vi "主板电池信息配置.vi"(2 "电池信息查看":string[][](table)) -> (0 "输出数组":string[][](array[string]), 1 "布尔":bool=TRUE)   [LabVIEW 2013]
panel:
  in  "整车CAN测试":bool
  in  "电池信息":T1
  in  "停止":bool
  in  "确定":bool
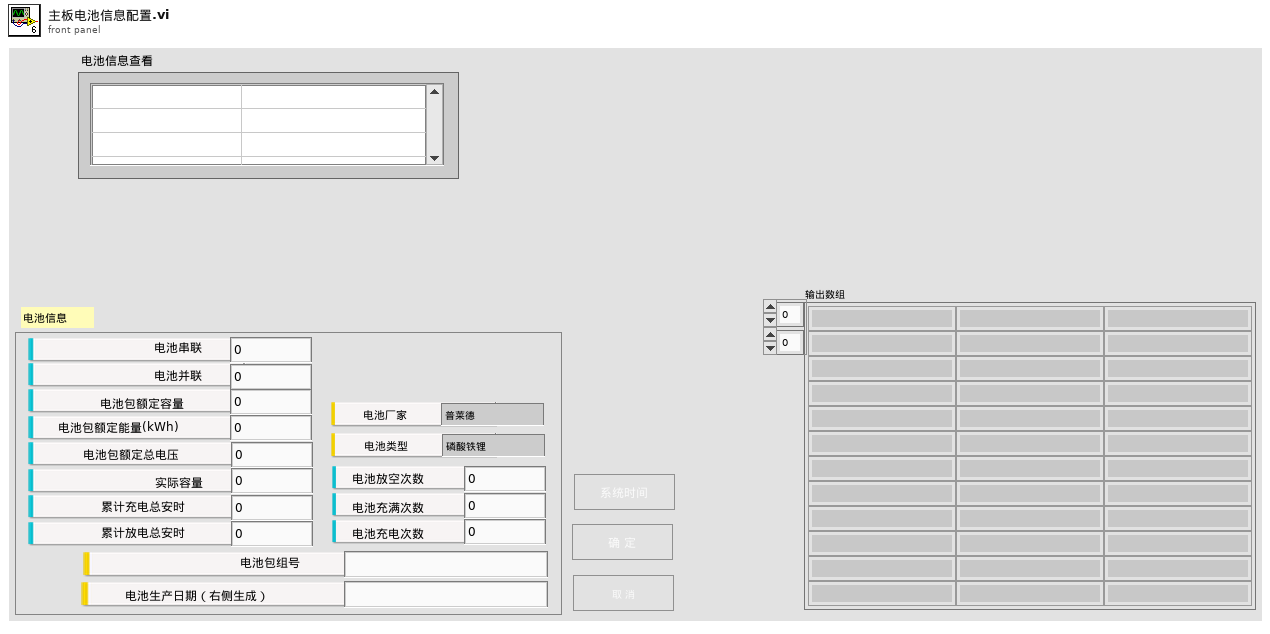
[diagram p1: front panel]
types:
  T1 = cluster{"电池串联":dbl, "电池并联":dbl, "电池包额定容量":dbl, "电池包额定能量(kWh)":dbl, "电池包额定总电压":dbl, "实际容量":dbl, "电池厂家":enum16{"普莱德", "盟固利", "CALB", "力神", "波士顿", "BAK"}, "电池类型":enum16{"磷酸铁锂", "锰酸锂", "三元材料", "铅酸", "镍氢", "钴酸锂", "聚合物锂离子", "钛酸锂", "其他电池"}, "累计充电总安时":dbl, "累计放电总安时":dbl, "电池放空次数":dbl, "电池充满次数":dbl, "电池充电次数":dbl, "电池生产日期（右侧生成）":string, "电池包组号":string}
  T2 = enum16{"磷酸铁锂", "锰酸锂", "三元材料", "铅酸", "镍氢", "钴酸锂", "聚合物锂离子", "钛酸锂", "其他电池"}
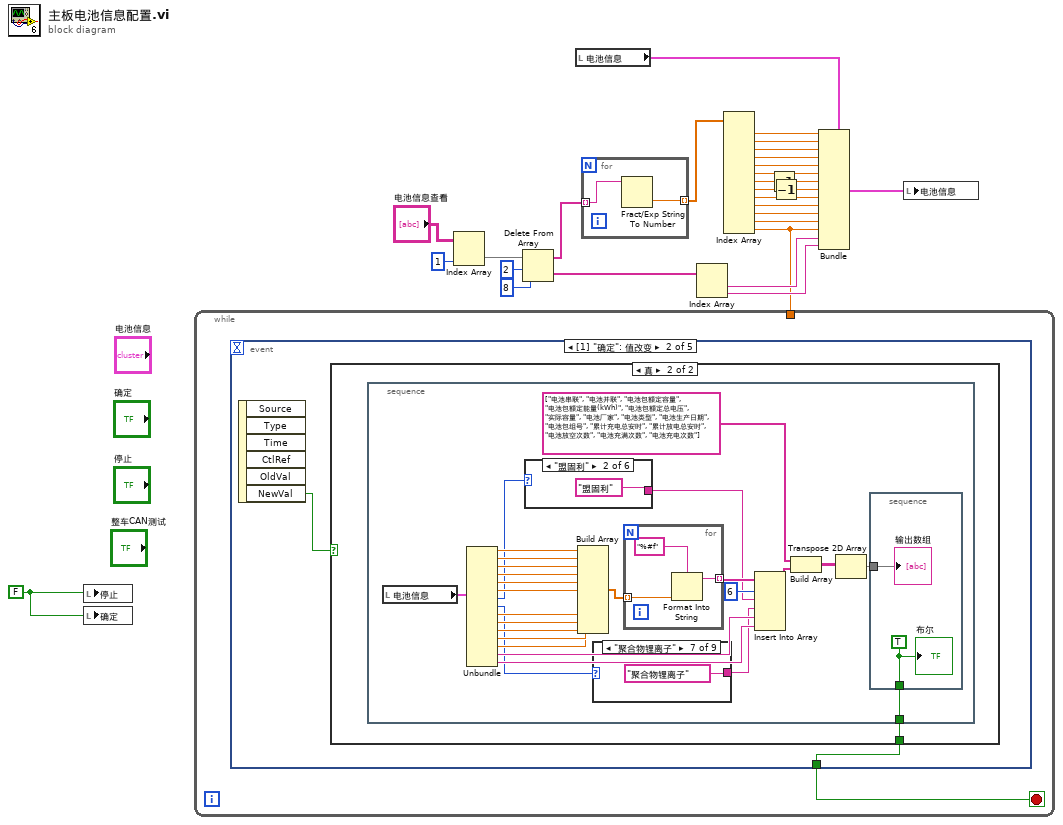
[diagram p0: block diagram]
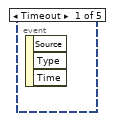
[diagram p2: hidden frame]
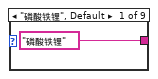
[diagram p4: hidden frame]
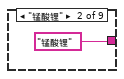
[diagram p5: hidden frame]
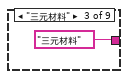
[diagram p6: hidden frame]
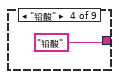
[diagram p7: hidden frame]
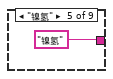
[diagram p8: hidden frame]
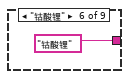
[diagram p9: hidden frame]
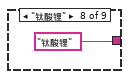
[diagram p10: hidden frame]
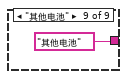
[diagram p11: hidden frame]
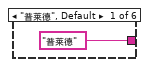
[diagram p12: hidden frame]
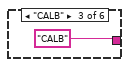
[diagram p13: hidden frame]
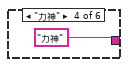
[diagram p14: hidden frame]
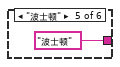
[diagram p15: hidden frame]
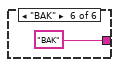
[diagram p16: hidden frame]
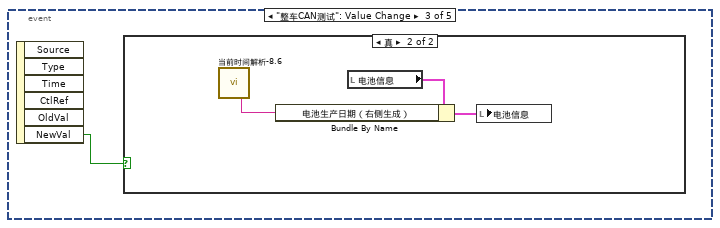
[diagram p17: hidden frame]
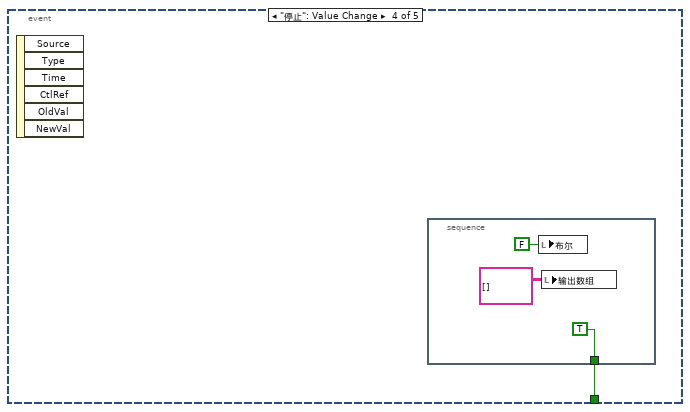
[diagram p19: hidden frame]
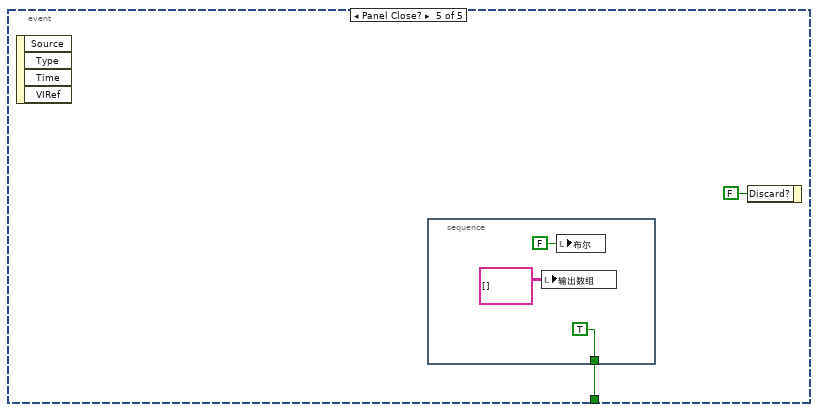
[diagram p20: hidden frame]
diagram:
  w28 = FALSE ("取消按钮")
  n1 = local write "停止"(w28) -> ()
  n2 = local write "确定"(w28) -> ()
  n3 = Index Array(array="电池信息查看", index (col)=1 ("禁用的索引 (列)")) -> (element=w25:string[])  [unwired: 1 in]
  n4 = Delete From Array(array=w25, length=2 ("长度"), index=8 ("索引")) -> (deleted portion=w19:string[], array with subset deleted=w22:string[])
  n5 = local read "电池信息"() -> (w21:T1)
  n6 = for {
    tunnel: w22 -> [w30] mode=indexing
    tunnel: [w29] -> w16 mode=indexing
    n7 = Fract/Exp String To Number(string=w30) -> (number=w29:dbl)  [unwired: 3 in, 1 out]
  }
  n8 = Index Array(array=w19) -> (element #1=w18:string, element #2=w17:string)  [unwired: 2 in]
  n9 = Index Array(array=w16) -> (element #1=w15:dbl, element #2=w14:dbl, element #3=w13:dbl, element #4=w12:dbl, element #5=w11:dbl, element #6=w10:dbl, element #7=w9:dbl, element #8=w8:dbl, element #9=w7:dbl, element #10=w6:dbl, element #11=w5:dbl, element #12=w4:dbl, element #13=w3:dbl)  [unwired: 13 in]
  n10 = while {
    tunnel: w3 -> [_]
    stop <- w31 stop-if-true
    n11 = event shown="[1] \"确定\": 值改变" {
      selector: _ -> [_ _ _ _ _]
      dyn-events: _ -> [_ _ _ _ _]
      timeout: _ -> [_ _ _ _ _]
      tunnel: [_ w32 _ w85 w90] -> w31
      event Timeout {
        n12 = event-data() -> ()  [unwired: 1 in, 3 out]
      }
      event "确定": Value Change {
        n13 = event-data() -> ("NewVal"=w33:bool)  [unwired: 1 in, 5 out]
        n14 = case shown="真" w33 {
          tunnel: [_ w34] -> w32
          frame False {
          }
          frame True {
            n15 = stacked-sequence {
              tunnel: [w41] -> w34
              frame #0 {
                n16 = local read "电池信息"() -> (w60:T1)
                n17 = Unbundle(w60) -> ("电池串联"=w59:dbl, "电池并联"=w58:dbl, "电池包额定容量"=w57:dbl, "电池包额定能量(kWh)"=w56:dbl, "电池包额定总电压"=w55:dbl, "实际容量"=w54:dbl, "电池厂家"=w38:enum16{"普莱德", "盟固利", "CALB", "力神", "波士顿", "BAK"}, "电池类型"=w37:T2, "累计充电总安时"=w53:dbl, "累计放电总安时"=w52:dbl, "电池放空次数"=w51:dbl, "电池充满次数"=w50:dbl, "电池充电次数"=w49:dbl, "电池生产日期（右侧生成）"=w40:string, "电池包组号"=w39:string)
                n18 = case shown="\"盟固利\"" w38 {
                  tunnel: ["普莱德" "盟固利" "CALB" "力神" "波士顿" "BAK"] -> w36
                  frame "普莱德", Default {
                  }
                  frame "盟固利" {
                  }
                  frame "CALB" {
                  }
                  frame "力神" {
                  }
                  frame "波士顿" {
                  }
                  frame "BAK" {
                  }
                }
                n19 = Build Array(w59, w58, w57, w56, w55, w54, w53, w52, w51, w50, w49) -> (w48:dbl[])
                n20 = case shown="\"聚合物锂离子\"" w37 {
                  tunnel: ["磷酸铁锂" "锰酸锂" "三元材料" "铅酸" "镍氢" "钴酸锂" "聚合物锂离子" "钛酸锂" "其他电池"] -> w35
                  frame "磷酸铁锂", Default {
                  }
                  frame "锰酸锂" {
                  }
                  frame "三元材料" {
                  }
                  frame "铅酸" {
                  }
                  frame "镍氢" {
                  }
                  frame "钴酸锂" {
                  }
                  frame "聚合物锂离子" {
                  }
                  frame "钛酸锂" {
                  }
                  frame "其他电池" {
                  }
                }
                n21 = for {
                  tunnel: w48 -> [w80] mode=indexing
                  tunnel: [w78] -> w47 mode=indexing
                  n22 = Format Into String(format string="%#f" ("格式字符串"), w80) -> (resulting string=w78:string)  [unwired: 2 in, 1 out]
                }
                n23 = Insert Into Array(array=w47, index=6 ("索引"), new element #1=w36, new element #2=w35, new element #3=w40, new element #4=w39) -> (w46:string[])
                n24 = Build Array(string[] ["电池串联", "电池并联", "电池包额定容量", "电池包额定能量(kWh)", "电池包额定总电压", "实际容量", "电池厂家", "电池类型", "电池生产日期", "电池包组号", "累计充电总安时", "累计放电总安时", "电池放空次数", "电池充满次数", "电池充电次数"], w46) -> (w44:string[][])
                n25 = Transpose 2D Array(2D array=w44) -> (transposed array=w43:string[][])
                n26 = stacked-sequence {
                  tunnel: w43 -> [w77]
                  tunnel: [w76] -> w41
                  frame #0 {
                    w76 = TRUE
                    "输出数组" <- w77
                    "布尔" <- w76
                  }
                }
              }
            }
          }
        }
      }
      event "整车CAN测试": Value Change {
        n27 = event-data() -> ("NewVal"=w81:bool)  [unwired: 1 in, 5 out]
        n28 = case shown="真" w81 {
          frame False {
          }
          frame True {
            n29 = call "当前时间解析-8.6.vi"() -> ("时间"=w82:string)  [unwired: 10 in, 9 out]
            n30 = local read "电池信息"() -> (w84:T1)
            n31 = Bundle By Name(cluster=w84, "电池生产日期（右侧生成）"=w82) -> (w83:T1)
            n32 = local write "电池信息"(w83) -> ()
          }
        }
      }
      event "停止": Value Change {
        n33 = event-data() -> ()  [unwired: 1 in, 6 out]
        n34 = stacked-sequence {
          tunnel: [TRUE] -> w85
          frame #0 {
            n35 = local write "布尔"(FALSE ("布尔")) -> ()
            n36 = local write "输出数组"(string[][] [] ("输出数组")) -> ()
          }
        }
      }
      event Panel Close? {
        n37 = event-data() -> ()  [unwired: 1 in, 4 out]
        n38 = stacked-sequence {
          tunnel: [TRUE] -> w90
          frame #0 {
            n39 = local write "输出数组"(string[][] [] ("输出数组")) -> ()
            n40 = local write "布尔"(FALSE ("布尔")) -> ()
          }
        }
        n41 = event-data("Discard?"=FALSE ("放弃？")) -> ()  [unwired: 1 in, 1 out]
      }
    }
  }
  n42 = Decrement(x=w9) -> (x-1=w2:dbl)
  n43 = Decrement(x=w8) -> (x-1=w1:dbl)
  n44 = Bundle(cluster=w21, "电池串联"=w15, "电池并联"=w14, "电池包额定容量"=w13, "电池包额定能量(kWh)"=w12, "电池包额定总电压"=w11, "实际容量"=w10, "电池厂家"=w2, "电池类型"=w1, "累计充电总安时"=w7, "累计放电总安时"=w6, "电池放空次数"=w5, "电池充满次数"=w4, "电池充电次数"=w3, "电池生产日期（右侧生成）"=w18, "电池包组号"=w17) -> (w20:T1)
  n45 = local write "电池信息"(w20) -> ()
